vi "Create enPassant Move.vi"(6 "enPassant target":T1={"File"=enum."d", "Rank"=enum."4"}, 9 "Destination":T1={"File"=enum."d", "Rank"=enum."4"}, 10 "Source":T1={"File"=enum."d", "Rank"=enum."4"}, 11 "Pawn":refnum<class "Pawn.lvclass">) -> (3 "enPassant out":refnum<class "enPassant.lvclass">)   [LabVIEW 2015, in "Chesslib.lvlib" / "enPassant.lvclass"]
uses:
  enPassant.lvclass
  typedef/Square.ctl
  typedef/File.ctl
  typedef/Rank.ctl
  Pieces/Pawn/Pawn.lvclass
  enPassant.lvclass/enPassant.ctl
  Move/Move.lvclass
  Chesslib.lvlib
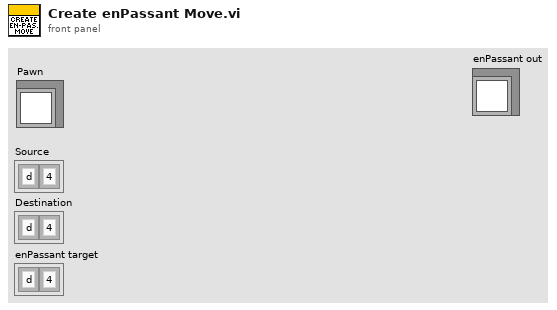
[diagram p1: front panel]
types:
  T1 = typedef "Chesslib.lvlib/Square.ctl" = cluster{"File":T2, "Rank":T3}
  T2 = typedef "Chesslib.lvlib/File.ctl" = enum8{"a", "b", "c", "d", "e", "f", "g", "h"}
  T3 = typedef "Chesslib.lvlib/Rank.ctl" = enum8{"1", "2", "3", "4", "5", "6", "7", "8"}
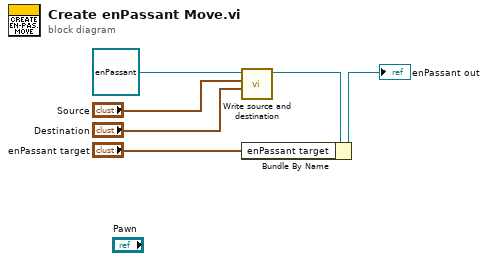
[diagram p0: block diagram]
diagram:
  n1 = call "Write source and destination.vi"("Destination"="Destination", "Source"="Source", "Move in"=refnum<class "enPassant.lvclass"> refnum ("enPassant in")) -> ("Move out"=w1:refnum<class "enPassant.lvclass">)  [unwired: 8 in]
  n2 = Bundle By Name(cluster=w1, "enPassant target"="enPassant target") -> (→"enPassant out":refnum<class "enPassant.lvclass">)
